vi "cycle_AsH3.vi"(2 "Debug Mode":bool, 3 "Elapsed Time (s)":dbl, 4 "State":enum16{"Edit", "Start", "Run", "End", "Idle"}(ring), 5 "Argument List In":string[](array[string])) -> (0 "Status Out":string, 1 "Argument List Out":string[](array[string]))   [LabVIEW 2011]
panel:
  in  "period (s)":dbl
  in  "flow rate (sccm)":dbl
  in  "# of cycles":dbl
  in  "Cancel":bool
  in  "Gas Source In":bool
  in  "OK":bool
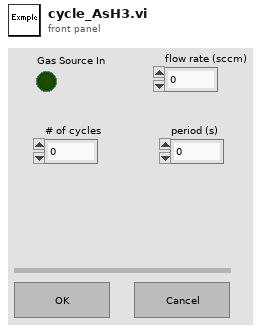
[diagram p1: front panel]
types:
  T1 = enum16{"Discrete", "Continuous", "Instantaneous"}
  T2 = enum32{"Invalid", "Default", "Floating", "Floating/Auto-Hide", "Modal"}
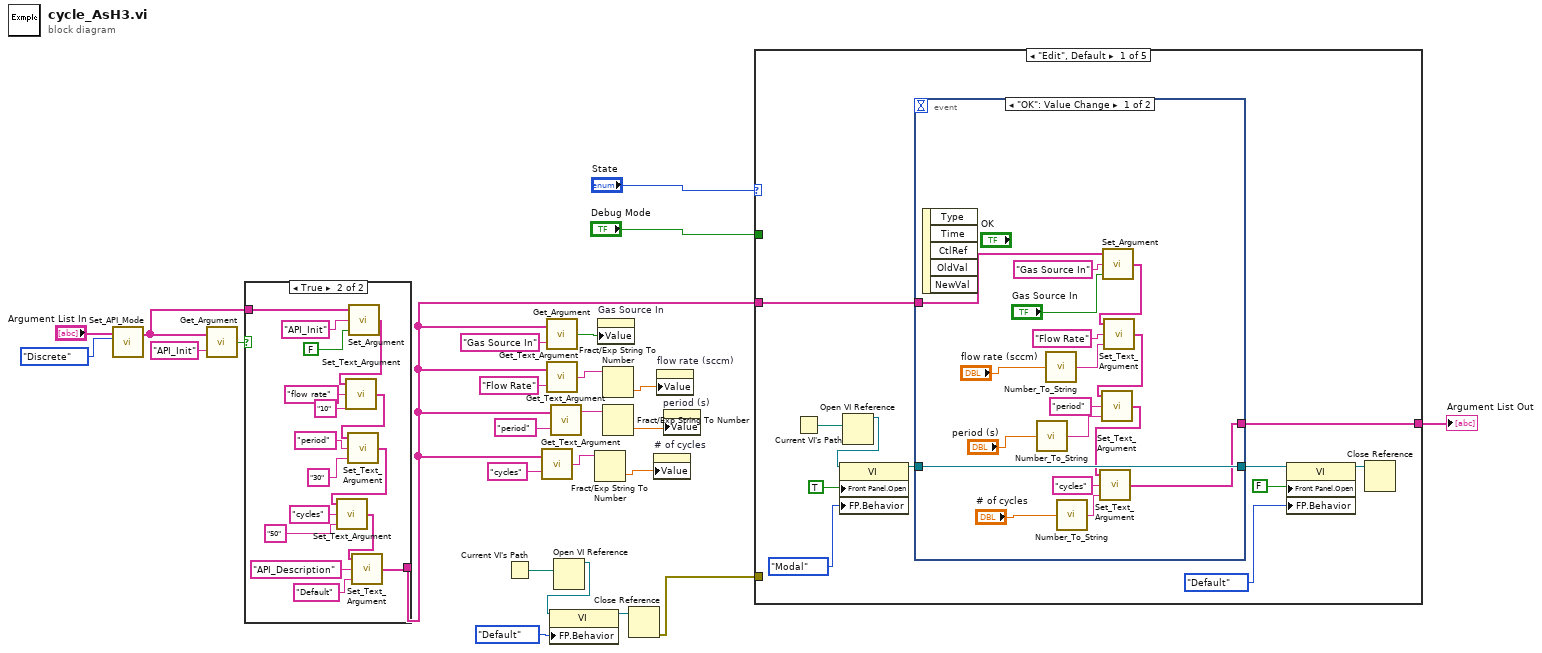
[diagram p0: block diagram]
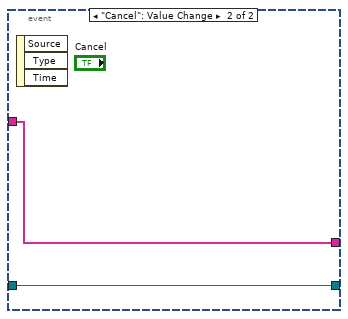
[diagram p3: hidden frame]
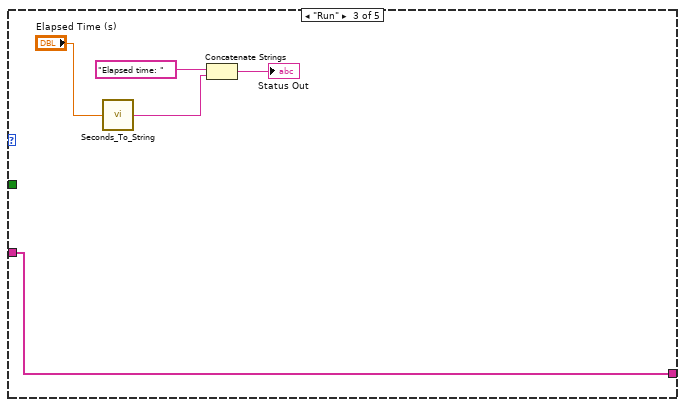
[diagram p5: hidden frame]
diagram:
  n1 = call "Set_API_Mode.vi"("API Mode"=T1."Discrete", "Argument List In"="Argument List In") -> ("Argument List Out"=w8:string[])  [unwired: 3 in]
  n2 = call "Get_Argument.vi"("Argument"="API_Init", "Argument List"=w8) -> ("Enabled"=w9:bool)
  n3 = case shown="True" w9 {
    tunnel: w8 -> [w26 w42]
    tunnel: [w26 w38] -> w4
    frame False {
    }
    frame True {
      n4 = call "Set_Argument.vi"("Enable"=FALSE, "Argument"="API_Init", "Argument List In"=w42) -> ("Argument List Out"=w30:string[])
      n5 = call "Set_Text_Argument.vi"("Text"="10", "Argument"="flow rate", "Argument List In"=w30) -> ("Argument List Out"=w29:string[])
      n6 = call "Set_Text_Argument.vi"("Text"="30", "Argument"="period", "Argument List In"=w29) -> ("Argument List Out"=w31:string[])
      n7 = call "Set_Text_Argument.vi"("Text"="50", "Argument"="cycles", "Argument List In"=w31) -> ("Argument List Out"=w35:string[])
      n8 = call "Set_Text_Argument.vi"("Text"="Default", "Argument"="API_Description", "Argument List In"=w35) -> ("Argument List Out"=w38:string[])
    }
  }
  n9 = Current VI's Path() -> (path=w19:path)
  n10 = call "Get_Text_Argument.vi"("Argument"="cycles", "Argument List"=w4) -> ("Text"=w6:string)
  n11 = call "Get_Argument.vi"("Argument"="Gas Source In", "Argument List"=w4) -> ("Enabled"=w21:bool)
  n12 = call "Get_Text_Argument.vi"("Argument"="Flow Rate", "Argument List"=w4) -> ("Text"=w7:string)
  n13 = call "Get_Text_Argument.vi"("Argument"="period", "Argument List"=w4) -> ("Text"=w14:string)
  n14 = Open VI Reference(vi path=w19) -> (vi reference=w18:refnum<vi>)  [unwired: 1 in, 5 out]
  n15 = property class="VI"(reference=w18, "FP.Behavior"=T2."Default" ("Front Panel Window:Behavior")) -> (reference out=w16:refnum<vi>)  [unwired: 1 in, 1 out]
  n16 = Fract/Exp String To Number(string=w6) -> (number=w1:dbl)  [unwired: 4 out]
  n17 = property on="Gas Source In" class="Bool (strict)"("Value"=w21) -> ()  [unwired: 2 in, 2 out]
  n18 = Fract/Exp String To Number(string=w7) -> (number=w3:dbl)  [unwired: 4 out]
  n19 = Fract/Exp String To Number(string=w14) -> (number=w2:dbl)  [unwired: 4 out]
  n20 = Close Reference(reference=w16) -> (error out=w15:errorcluster)  [unwired: 1 in]
  n21 = property on="# of cycles" class="DigNum (strict)"("Value"=w1) -> ()  [unwired: 2 in, 2 out]
  n22 = property on="flow rate (sccm)" class="DigNum (strict)"("Value"=w3) -> ()  [unwired: 2 in, 2 out]
  n23 = property on="period (s)" class="DigNum (strict)"("Value"=w2) -> ()  [unwired: 2 in, 2 out]
  n24 = case shown="\"Edit\", Default" "State" {
    tunnel: [w53 w73 w74 w79 w80] -> w24
    tunnel: w4 -> [w52 w73 w74 w79 w80]
    tunnel: "Debug Mode" -> [_ _ _ _ _]
    tunnel: w15 -> [_ _ _ _ _]
    frame "Edit", Default {
      n25 = Current VI's Path() -> (path=w47:path)
      n26 = Open VI Reference(vi path=w47) -> (vi reference=w46:refnum<vi>)  [unwired: 1 in, 5 out]
      n27 = property class="VI"(reference=w46, "Front Panel.Open"=TRUE ("Front Panel Window:Open"), "FP.Behavior"=T2."Modal" ("Front Panel Window:Behavior")) -> (reference out=w50:refnum<vi>)  [unwired: 1 in, 1 out]
      n28 = event shown="[0] \"OK\": Value Change" {
        selector: _ -> [_ _]
        dyn-events: _ -> [_ _]
        timeout: _ -> [_ _]
        tunnel: w52 -> [w67 w71]
        tunnel: [w59 w71] -> w53
        tunnel: [w65 w72] -> w49
        tunnel: w50 -> [w65 w72]
        event "OK": Value Change {
          n29 = event-data() -> ()  [unwired: 6 out]
          n30 = call "Number_To_String.vi"("Number"="period (s)") -> ("String"=w62:string)
          n31 = call "Number_To_String.vi"("Number"="flow rate (sccm)") -> ("String"=w60:string)
          n32 = call "Number_To_String.vi"("Number"="# of cycles") -> ("String"=w58:string)
          n33 = call "Set_Argument.vi"("Enable"="Gas Source In", "Argument"="Gas Source In", "Argument List In"=w67) -> ("Argument List Out"=w66:string[])
          n34 = call "Set_Text_Argument.vi"("Text"=w60, "Argument"="Flow Rate" ("Text"), "Argument List In"=w66) -> ("Argument List Out"=w63:string[])
          n35 = call "Set_Text_Argument.vi"("Text"=w62, "Argument"="period", "Argument List In"=w63) -> ("Argument List Out"=w56:string[])
          n36 = call "Set_Text_Argument.vi"("Text"=w58, "Argument"="cycles", "Argument List In"=w56) -> ("Argument List Out"=w59:string[])
        }
        event "Cancel": Value Change {
          n37 = event-data() -> ()  [unwired: 4 out]
        }
      }
      n38 = property class="VI"(reference=w49, "Front Panel.Open"=FALSE ("Front Panel Window:Open"), "FP.Behavior"=T2."Default" ("Front Panel Window:Behavior")) -> (reference out=w43:refnum<vi>)  [unwired: 1 in, 1 out]
      n39 = Close Reference(reference=w43) -> ()  [unwired: 1 in, 1 out]
    }
    frame "Start" {
    }
    frame "Run" {
      n40 = call "Seconds_To_String.vi"("Seconds"="Elapsed Time (s)") -> ("Output String"=w76:string)
      n41 = Concatenate Strings("Elapsed time: " ("string"), w76) -> (→"Status Out":string)
    }
    frame "End" {
    }
    frame "Idle" {
    }
  }
  "Argument List Out" <- w24
